vi "VMUIAsync_Read-only.vi"(10 "SubPanelRef":refnum<vi>, 11 "VariableManagerRef in":refnum<vi>) -> ()   [LabVIEW 2013]
doc: "Asynchronously call VMUI.vi with the given input. The caller process will not be blocked."
uses:
  VariableManager/VariableManager.lvclass
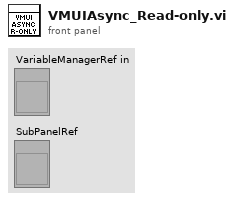
[diagram p1: front panel]
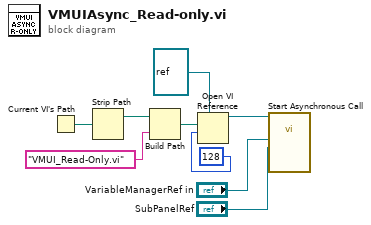
[diagram p0: block diagram]
diagram:
  n1 = Current VI's Path() -> (path=w7:path)
  n2 = Strip Path(path=w7) -> (stripped path=w8:path)  [unwired: 1 out]
  n3 = Build Path(base path=w8, name or relative path="VMUI_Read-Only.vi") -> (appended path=w6:path)
  n4 = Open VI Reference(type specifier VI Refnum (for type only)=refnum<vi> refnum, vi path=w6, options=128) -> (vi reference=w2:refnum<vi>)  [unwired: 3 in, 1 out]
  n5 = call-by-ref "Start Asynchronous Call"(reference=w2, "SubPanelRef"="SubPanelRef", "VariableManagerRef in"="VariableManagerRef in") -> ()  [unwired: 10 in, 3 out]
